vi "GT Pvt Table Complete.vi"(0 "cardNum":i16, 1 "tableId":i16, 2 "count":i32, 3 "pTime":dbl[](array[numeric]), 4 "pPos":dbl[](array[numeric]), 5 "pA":dbl, 6 "pB":dbl, 7 "error in (no error)":errorcluster caption="错误输入（无错误）", 8 "pC":dbl, 9 "velBegin":dbl, 10 "velEnd":dbl) -> (18 "pC out":dbl, 20 "function return":i16, 23 "pTime out":dbl[](array[numeric]), 24 "pPos out":dbl[](array[numeric]), 25 "pA out":dbl, 26 "pB out":dbl, 27 "error out":errorcluster caption="错误输出")   [LabVIEW 2014, in "gts.lvlib"]
doc: "GT_API GT_PvtTableComplete(short cardNum,short tableId,long count,double *pTime,double *pPos,double *pA,double *pB,double *pC,double velBegin=0,double velEnd=0);"
uses:
  gts.lvlib
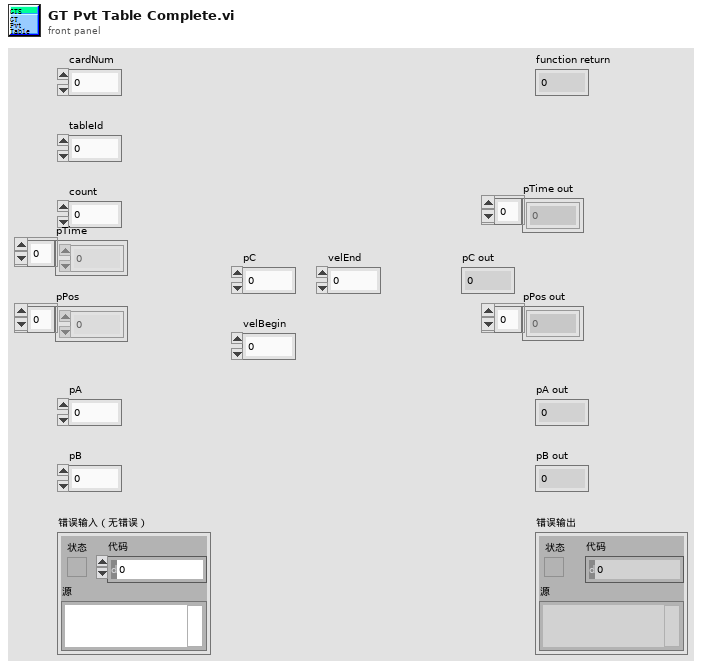
[diagram p1: front panel]
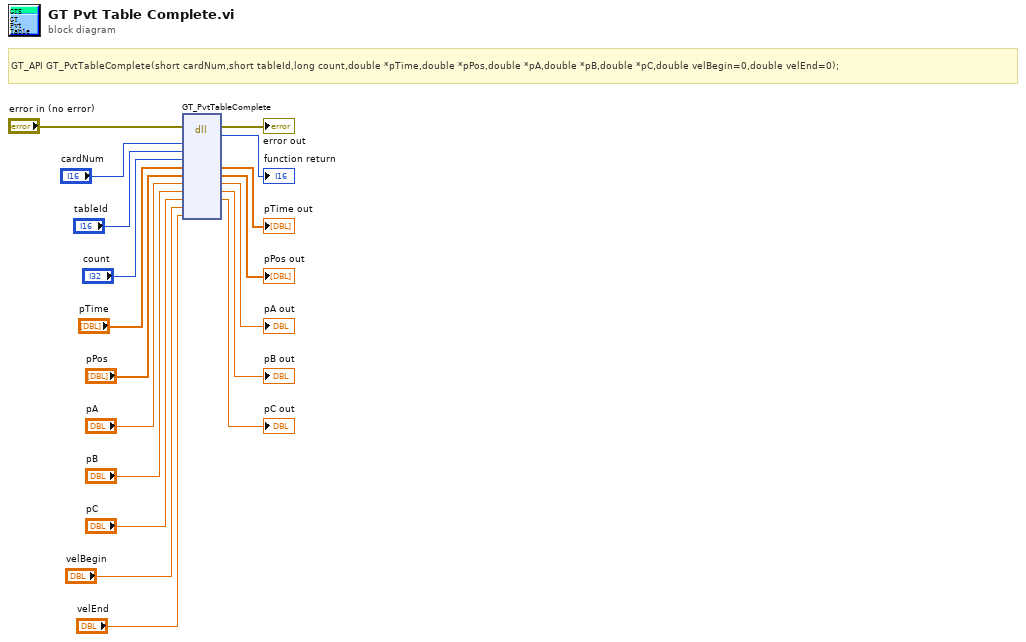
[diagram p0: block diagram]
diagram:
  # "GT_API GT_PvtTableComplete(short cardNum,short tableId,long count,double *pTime,double *pPos,double *pA,double *pB,double *pC,double velBegin=0,double velEnd=0);"
  n1 = dll-call lib="PTH2habs D固高科技资料GTS控制卡GTS卡18年上半年资料dllVC32bit\nmulti_cardgts.*" fn="GT_PvtTableComplete"(error in="error in (no error)", "cardNum"="cardNum", "tableId"="tableId", "count"="count", "pTime"="pTime", "pPos"="pPos", "pA"="pA", "pB"="pB", "pC"="pC", "velBegin"="velBegin", "velEnd"="velEnd") -> (error out=→"error out":errorcluster, "返回类型"=→"function return":i16, "pTime"=→"pTime out":dbl[], "pPos"=→"pPos out":dbl[], "pA"=→"pA out":dbl, "pB"=→"pB out":dbl, "pC"=→"pC out":dbl)  [unwired: 7 in, 1 out]
